vi "Prober_ProbeTouchdown.vi"(8 "error in (no error)":errorcluster, 11 "ProbeStationControl in":refnum<class "ProbeStationControl.lvclass">) -> (0 "error out":errorcluster, 1 "previous Z [µm]":i32, 2 "Z [µm]":i32, 3 "ProbeStationControl out":refnum<class "ProbeStationControl.lvclass">)   [LabVIEW 2019, in "ProbeStationControl.lvclass"]
uses:
  ProbeStationControl.lvclass
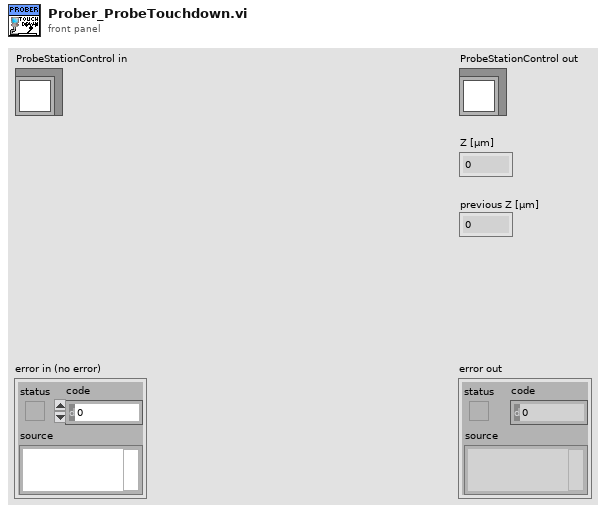
[diagram p1: front panel]
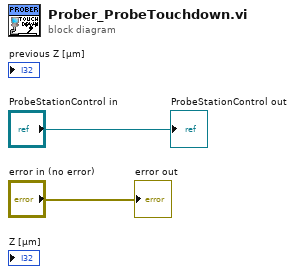
[diagram p0: block diagram]
diagram:
  "error out" <- "error in (no error)"
  "ProbeStationControl out" <- "ProbeStationControl in"
